vi "ATF-Pump-Sequence Control FGV.vi"(7 "Enum":enum16{"Write", "Read"}(ring)=enum."Read", 8 "error in":errorcluster, 10 "SEQUENCE CONTROL":T1) -> (0 "error out":errorcluster, 2 "SEQUENCE CONTROL OUT":T1)   [LabVIEW 2022 SP3]
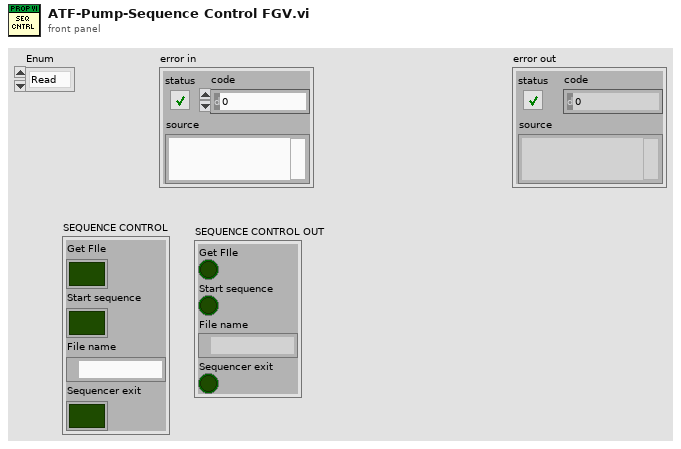
[diagram p1: front panel]
types:
  T1 = cluster{"Get FIle":bool, "Start sequence":bool, "File name ":path, "Sequencer exit":bool}
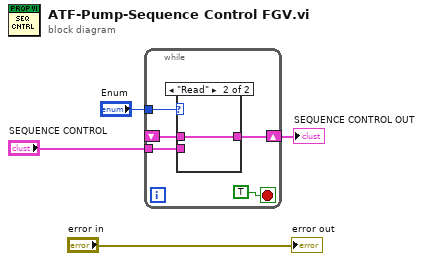
[diagram p0: block diagram]
diagram:
  n1 = while {
    tunnel: "Enum" -> [w9]
    tunnel: "SEQUENCE CONTROL" -> [w7]
    shift-right: [w6] -> w1
    shift-left: _ -> [w5]
    stop <- TRUE stop-if-true
    n2 = case shown="\"Read\"" w9 {
      tunnel: w7 -> [w10 _]
      tunnel: [w10 w11] -> w6
      tunnel: w5 -> [_ w11]
      frame "Write", Default {
      }
      frame "Read" {
      }
    }
  }
  "SEQUENCE CONTROL OUT" <- w1
  "error out" <- "error in"
